vi "SetParameter.vi"(8 "error in (no error)":errorcluster, 10 "SetParameter":T1, 11 "ChromaAcLoad in":refnum<class "ChromaAcLoad.lvclass">) -> (0 "error out":errorcluster, 2 "StatusUpdates":string[](array[string]), 3 "ChromaAcLoad out":refnum<class "ChromaAcLoad.lvclass">)   [LabVIEW 2018, in "AcPwrPlugins.lvlib" / "ChromaAcLoad.lvclass"]
uses:
  ChromaAcLoad.lvclass
  AcPwrBaseClass/TypeDefs/SetParameterInputs.ctl
  TypeDefs/RangeCheck.ctl
  AcPwrBaseClass/AcPwrBase.lvclass
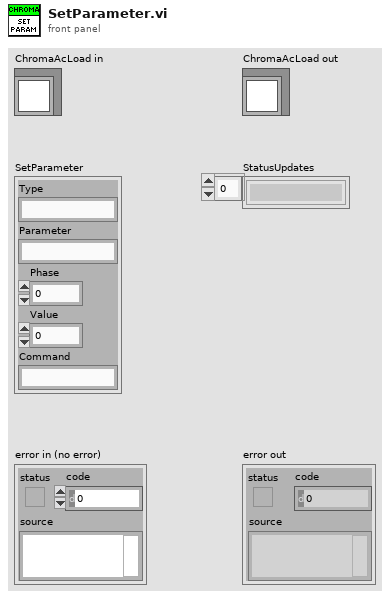
[diagram p1: front panel]
types:
  T1 = typedef "AcPwrPlugins.lvlib/AcPwrBase.lvclass/SetParameterInputs.ctl" = cluster{"Type":string, "Parameter":string, "Phase":i32, "Value":dbl, "Command":string}
  T2 = enum16{"Constant Voltage (DC)", "Constant Power (DC)", "Constant Power (AC)", "Constant Current (DC)", "Constant Current (AC)", "Constant Resistance (DC)", "Constant Resistance (AC)", "Rectified Mode (DC)", "Inrush (AC)", "RLC CP (AC)", "RLC (AC)"}
  T3 = cluster{"Handle":string, "Name":string, "Phase Select":i32, "Instrument Options":string, "id query (T)":bool, "reset device (T)":bool, "Load Short Circuited":bool, "Line Synchronization":bool, "Load Current (A/Arms)":dbl, "Load Voltage (V/Vrms)":dbl, "Load Power (W)":dbl, "Load Resistance (Ohms)":dbl, "Load Current Peak Limit (A)":dbl, "Load Current Limit (A/Arms)":dbl, "Load Power Limit (W)":dbl, "Synch Frequency (Hz)":dbl, "Priority":enum16{"CF Only", "PF Only", "Both (CF)", "Both (PF)"}, "Crest Factor":dbl, "Power Factor":dbl, "Slew Rate":cluster{"Rise Slew Rate (A/ms)":i32, "Fall Slew Rate (A/ms)":i32}, "LC/RLC Mode":cluster{"Capacitance (uF)":i32, "Inductance (uH)":i32, "Series Resistance (Ohm)":dbl, "Parallel Resistance (Ohm)":dbl}, "Timing":cluster{"TimingOn":enum16{""}, "Hours":u32, "Minutes":u32, "Seconds":dbl, "CutoffVoltage":dbl}, "Connected":bool}[]
  T4 = cluster{"Handle":string, "Name":string, "Phase Select":i32, "Instrument Options":string, "id query (T)":bool, "reset device (T)":bool, "Load Short Circuited":bool, "Line Synchronization":bool, "Load Current (A/Arms)":dbl, "Load Voltage (V/Vrms)":dbl, "Load Power (W)":dbl, "Load Resistance (Ohms)":dbl, "Load Current Peak Limit (A)":dbl, "Load Current Limit (A/Arms)":dbl, "Load Power Limit (W)":dbl, "Synch Frequency (Hz)":dbl, "Priority":enum16{"CF Only", "PF Only", "Both (CF)", "Both (PF)"}, "Crest Factor":dbl, "Power Factor":dbl, "Slew Rate":cluster{"Rise Slew Rate (A/ms)":i32, "Fall Slew Rate (A/ms)":i32}, "LC/RLC Mode":cluster{"Capacitance (uF)":i32, "Inductance (uH)":i32, "Series Resistance (Ohm)":dbl, "Parallel Resistance (Ohm)":dbl}, "Timing":cluster{"TimingOn":enum16{""}, "Hours":u32, "Minutes":u32, "Seconds":dbl, "CutoffVoltage":dbl}, "Connected":bool}
  T5 = typedef "AcPwrPlugins.lvlib/ChromaAcLoad.lvclass/RangeCheck.ctl" = enum16{"Power", "Power Limit", "Current", "Current Peak", "Current Limit", "Voltage", "AC Resistance", "DC Resistance", "Frequency", "Crest Factor", "Power Factor", "RLC Power Factor", "Rise Slew Rate", "Fall Slew Rate", "Capacitance", "Inductance", "Parallel Resistance", "Series Resistance"}[]
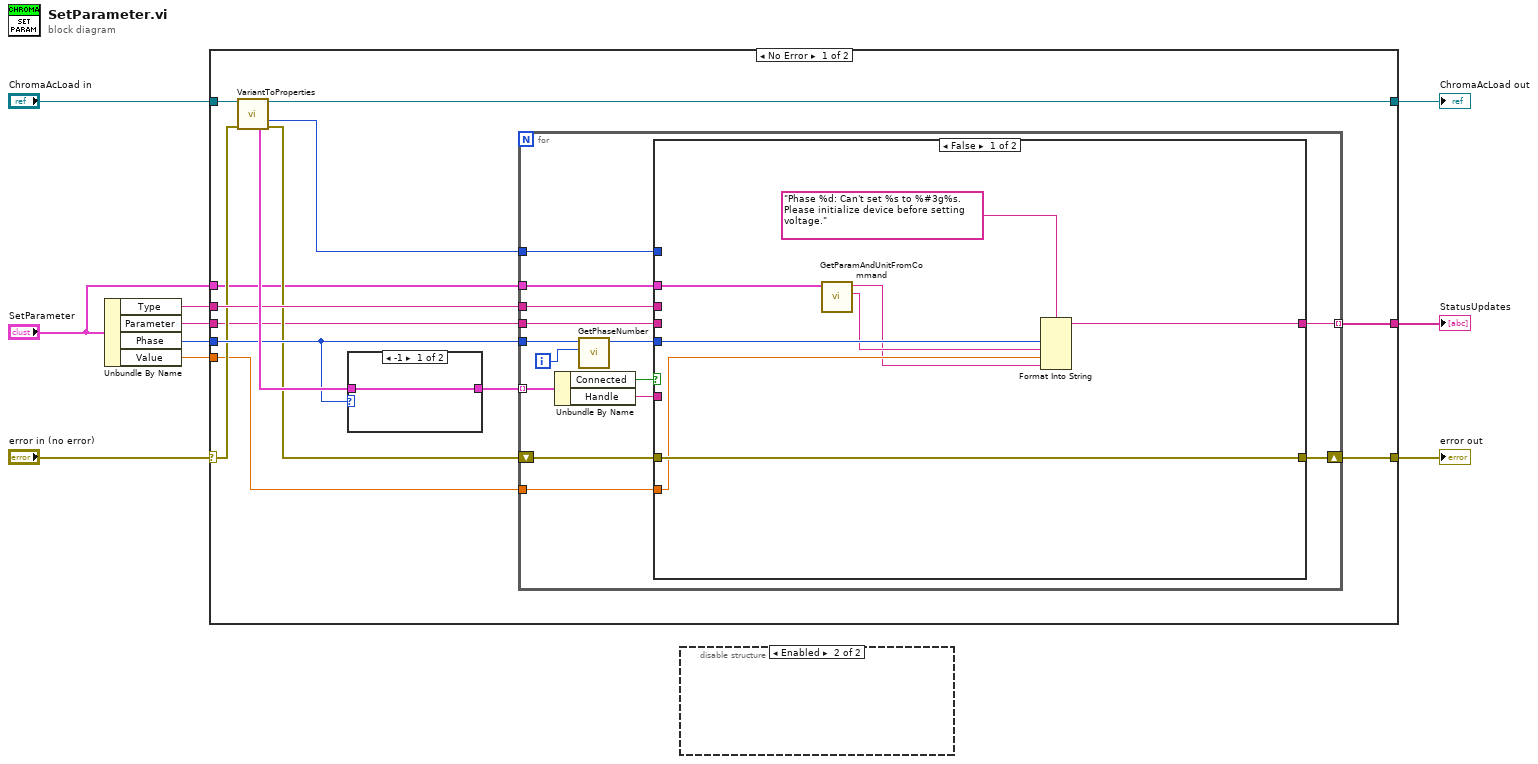
[diagram p0: block diagram]
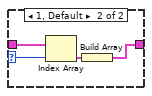
[diagram p2: hidden frame]
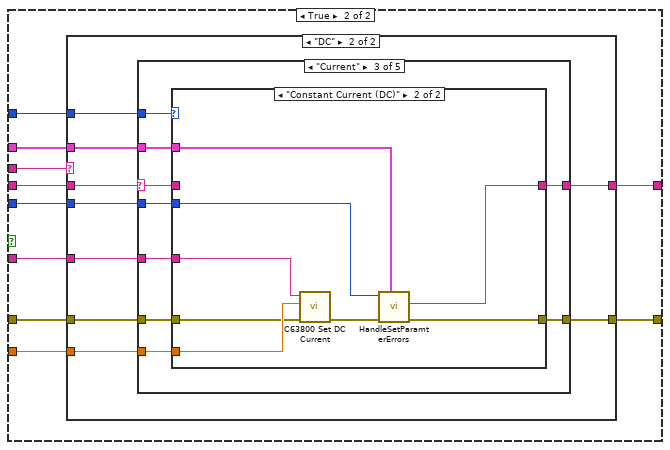
[diagram p3: hidden frame]
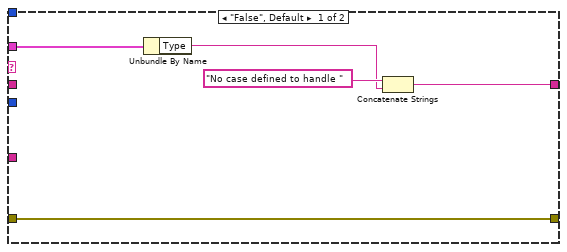
[diagram p4: hidden frame]
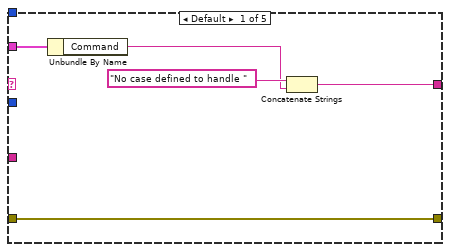
[diagram p5: hidden frame]
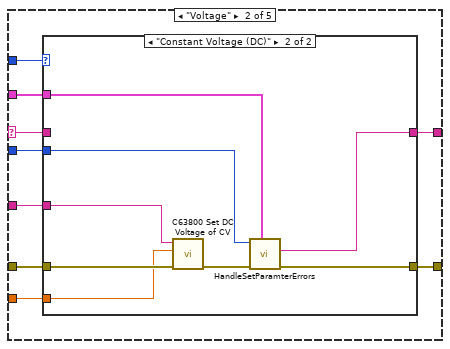
[diagram p6: hidden frame]
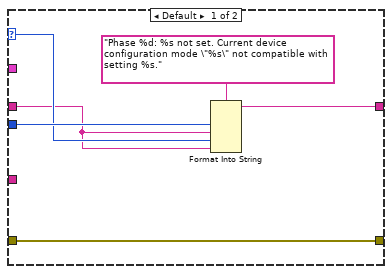
[diagram p7: hidden frame]
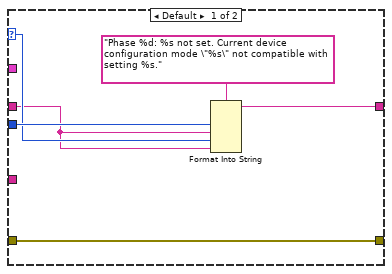
[diagram p8: hidden frame]
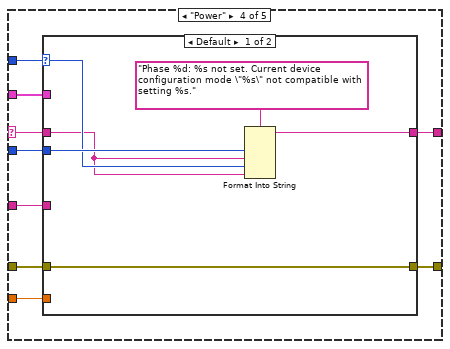
[diagram p9: hidden frame]
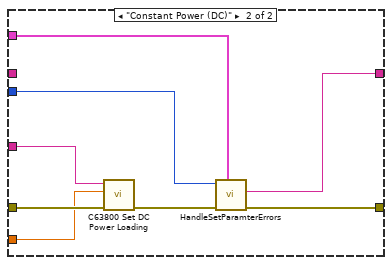
[diagram p10: hidden frame]
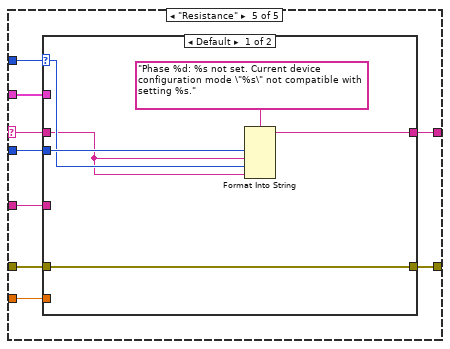
[diagram p11: hidden frame]
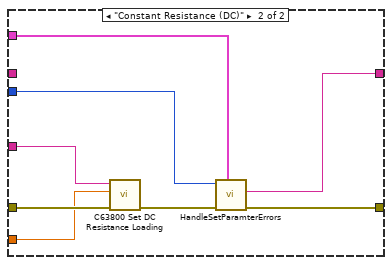
[diagram p12: hidden frame]
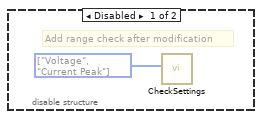
[diagram p14: hidden frame]
diagram:
  n1 = Unbundle By Name("SetParameter") -> ("Type"=w3:string, "Parameter"=w2:string, "Phase"=w5:i32, "Value"=w4:dbl)
  n2 = case shown="No Error" "error in (no error)" {
    selector: "error in (no error)" -> [w16 w174]
    tunnel: "ChromaAcLoad in" -> [w24 w173]
    tunnel: [w23 w173] -> w9
    tunnel: w5 -> [w19 _]
    tunnel: [w18 _] -> w8
    tunnel: w3 -> [w17 _]
    tunnel: [w14 w174] -> w6
    tunnel: w4 -> [w13 _]
    tunnel: w2 -> [w12 _]
    tunnel: "SetParameter" -> [w11 _]
    frame No Error {
      n3 = call "VariantToProperties.vi"("ChromaAcLoad"=w24, "error in (no error)"=w16) -> ("ChromaAcLoad"=w23:refnum<class "ChromaAcLoad.lvclass">, "Configuration Mode"=w20:T2, "Phases"=w22:T3, "error out"=w15:errorcluster)  [unwired: 7 in, 3 out]
      n4 = case shown="-1" w19 {
        selector: w19 -> [_ w26]
        tunnel: w22 -> [w25 w29]
        tunnel: [w25 w27] -> w21
        frame -1 {
        }
        frame 1, Default {
          n5 = Index Array(array=w29, index=w26) -> (element=w28:T4)
          n6 = Build Array(w28) -> (w27:T3)
        }
      }
      n7 = for {
        tunnel: w21 -> [w43] mode=indexing
        shift-right: [w41] -> w14
        shift-left: w15 -> [w42]
        tunnel: w13 -> [w38]
        tunnel: w20 -> [w37]
        tunnel: w19 -> [w35]
        tunnel: [w33] -> w18 mode=indexing
        tunnel: w17 -> [w32]
        tunnel: w12 -> [w31]
        tunnel: w11 -> [w30]
        i -> [w36]
        n8 = Unbundle By Name(w43) -> ("Connected"=w40:bool, "Handle"=w39:string)
        n9 = call "GetPhaseNumber.vi"("Loop Counter"=w36, "Phase(-1, all) in"=w35) -> ("Phase(-1, all) out"=w34:i32)  [unwired: 9 in]
        n10 = case shown="False" w40 {
          tunnel: w42 -> [w51 w61]
          tunnel: [w51 w60] -> w41
          tunnel: w39 -> [_ w59]
          tunnel: w38 -> [w45 w58]
          tunnel: w37 -> [_ w57]
          tunnel: w34 -> [w50 w56]
          tunnel: [w48 w55] -> w33
          tunnel: w32 -> [_ w54]
          tunnel: w31 -> [_ w53]
          tunnel: w30 -> [w47 w52]
          frame False {
            n11 = call "GetParamAndUnitFromCommand.vi"("SetParameter"=w47) -> ("Parameter"=w46:string, "Unit Label"=w44:string)  [unwired: 9 in]
            n12 = Format Into String(format string="Phase %d: Can't set %s to %#3g%s. Please initialize device before setting voltage.", w50, w46, w45, w44) -> (resulting string=w48:string)  [unwired: 2 in, 1 out]
          }
          frame True {
            n13 = case shown="\"DC\"" w54 {
              tunnel: w61 -> [w62 w75]
              tunnel: [w62 w74] -> w60
              tunnel: w59 -> [_ w73]
              tunnel: w58 -> [_ w72]
              tunnel: w57 -> [_ w71]
              tunnel: w56 -> [_ w70]
              tunnel: [w63 w69] -> w55
              tunnel: w53 -> [_ w68]
              tunnel: w52 -> [w64 w67]
              frame "False", Default {
                n14 = Unbundle By Name(w64) -> ("Type"=w65:string)
                n15 = Concatenate Strings("No case defined to handle " ("string"), w65) -> (w63:string)
              }
              frame "DC" {
                n16 = case shown="\"Current\"" w68 {
                  selector: w68 -> [_ w82 w104 w127 w150]
                  tunnel: w75 -> [w80 w89 w112 w135 w158]
                  tunnel: [w80 w88 w111 w134 w157] -> w74
                  tunnel: w73 -> [_ w87 w110 w133 w156]
                  tunnel: w72 -> [_ w86 w109 w132 w155]
                  tunnel: w71 -> [_ w85 w108 w131 w154]
                  tunnel: w70 -> [_ w84 w107 w130 w153]
                  tunnel: [w79 w83 w106 w129 w152] -> w69
                  tunnel: w67 -> [w77 w81 w105 w128 w151]
                  frame Default {
                    n17 = Unbundle By Name(w77) -> ("Command"=w76:string)
                    n18 = Concatenate Strings("No case defined to handle " ("string"), w76) -> (w79:string)
                  }
                  frame "Voltage" {
                    n19 = case shown="\"Constant Voltage (DC)\"" w85 {
                      selector: w85 -> [w91 _]
                      tunnel: w89 -> [w95 w103]
                      tunnel: [w95 w100] -> w88
                      tunnel: w87 -> [_ w102]
                      tunnel: w86 -> [_ w98]
                      tunnel: w84 -> [w93 w99]
                      tunnel: [w92 w97] -> w83
                      tunnel: w81 -> [_ w96]
                      tunnel: w82 -> [w90 _]
                      frame Default {
                        n20 = Format Into String(format string="Phase %d: %s not set. Current device configuration mode \"%s\" not compatible with setting %s.", w93, w90, w91, w90) -> (resulting string=w92:string)  [unwired: 2 in, 1 out]
                      }
                      frame "Constant Voltage (DC)" {
                        n21 = call <instrlib>:"C63800 Set DC Voltage of CV.vi"("error in (no error)"=w103, "SetDCVoltageofCV"=w98, "Instrument Handle"=w102) -> ("error out"=w101:errorcluster)  [unwired: 7 in, 1 out]
                        n22 = call "HandleSetParamterErrors.vi"("SetParameter"=w96, "error in (no error)"=w101, "Phase"=w99) -> ("error IO"=w100:errorcluster, "Status Update"=w97:string)  [unwired: 7 in]
                      }
                    }
                  }
                  frame "Current" {
                    n23 = case shown="\"Constant Current (DC)\"" w108 {
                      selector: w108 -> [w114 _]
                      tunnel: w112 -> [w118 w120]
                      tunnel: [w118 w126] -> w111
                      tunnel: w110 -> [_ w122]
                      tunnel: w109 -> [_ w121]
                      tunnel: w107 -> [w116 w125]
                      tunnel: [w115 w124] -> w106
                      tunnel: w105 -> [_ w123]
                      tunnel: w104 -> [w113 _]
                      frame Default {
                        n24 = Format Into String(format string="Phase %d: %s not set. Current device configuration mode \"%s\" not compatible with setting %s.", w116, w113, w114, w113) -> (resulting string=w115:string)  [unwired: 2 in, 1 out]
                      }
                      frame "Constant Current (DC)" {
                        n25 = call <instrlib>:"C63800 Set DC Current.vi"("error in (no error)"=w120, "Set DC Current"=w121, "Instrument Handle"=w122) -> ("error out"=w119:errorcluster)  [unwired: 7 in, 1 out]
                        n26 = call "HandleSetParamterErrors.vi"("SetParameter"=w123, "error in (no error)"=w119, "Phase"=w125) -> ("error IO"=w126:errorcluster, "Status Update"=w124:string)  [unwired: 7 in]
                      }
                    }
                  }
                  frame "Power" {
                    n27 = case shown="Default" w131 {
                      selector: w131 -> [w137 _]
                      tunnel: w135 -> [w141 w145]
                      tunnel: [w141 w149] -> w134
                      tunnel: w133 -> [_ w143]
                      tunnel: w132 -> [_ w142]
                      tunnel: w130 -> [w139 w148]
                      tunnel: [w138 w147] -> w129
                      tunnel: w128 -> [_ w146]
                      tunnel: w127 -> [w136 _]
                      frame Default {
                        n28 = Format Into String(format string="Phase %d: %s not set. Current device configuration mode \"%s\" not compatible with setting %s.", w139, w136, w137, w136) -> (resulting string=w138:string)  [unwired: 2 in, 1 out]
                      }
                      frame "Constant Power (DC)" {
                        n29 = call <instrlib>:"C63800 Set DC Power Loading.vi"("error in (no error)"=w145, "DC Power Loading"=w142, "Instrument Handle"=w143) -> ("error out"=w144:errorcluster)  [unwired: 7 in, 1 out]
                        n30 = call "HandleSetParamterErrors.vi"("SetParameter"=w146, "error in (no error)"=w144, "Phase"=w148) -> ("error IO"=w149:errorcluster, "Status Update"=w147:string)  [unwired: 7 in]
                      }
                    }
                  }
                  frame "Resistance" {
                    n31 = case shown="Default" w154 {
                      selector: w154 -> [w160 _]
                      tunnel: w158 -> [w164 w168]
                      tunnel: [w164 w172] -> w157
                      tunnel: w156 -> [_ w166]
                      tunnel: w155 -> [_ w165]
                      tunnel: w153 -> [w162 w171]
                      tunnel: [w161 w170] -> w152
                      tunnel: w151 -> [_ w169]
                      tunnel: w150 -> [w159 _]
                      frame Default {
                        n32 = Format Into String(format string="Phase %d: %s not set. Current device configuration mode \"%s\" not compatible with setting %s.", w162, w159, w160, w159) -> (resulting string=w161:string)  [unwired: 2 in, 1 out]
                      }
                      frame "Constant Resistance (DC)" {
                        n33 = call <instrlib>:"C63800 Set DC Resistance Loading.vi"("error in (no error)"=w168, "DC Resistance Loading"=w165, "Instrument Handle"=w166) -> ("error out"=w167:errorcluster)  [unwired: 7 in, 1 out]
                        n34 = call "HandleSetParamterErrors.vi"("SetParameter"=w169, "error in (no error)"=w167, "Phase"=w171) -> ("error IO"=w172:errorcluster, "Status Update"=w170:string)  [unwired: 7 in]
                      }
                    }
                  }
                }
              }
            }
          }
        }
      }
    }
    frame Error {
    }
  }
  "error out" <- w6
  "ChromaAcLoad out" <- w9
  "StatusUpdates" <- w8
  n35 = disable-structure shown="Enabled" {
    frame Disabled {
      w176 = T5 [enum."Voltage", enum."Current Peak"] items=["Power", "Power Limit", "Current", "Current Peak", "Current Limit", "Voltage", "AC Resistance", "DC Resistance", "Frequency", "Crest Factor", "Power Factor", "RLC Power Factor", "Rise Slew Rate", "Fall Slew Rate", "Capacitance", "Inductance", "Parallel Resistance", "Series Resistance"] ("RangeCheck")
      # "Add range check after modification"
      n36 = call-dynamic "CheckSettings.vi"("RangeCheck"=w176) -> ("error in (no error)"=w175:errorcluster)  [unwired: 7 in, 2 out]
    }
    frame Enabled {
    }
  }
